vi "Module ID.vi"(11 "Config Monitor Module in":refnum<class "Config Monitor Module.lvclass">) -> (2 "Module ID":string)   [LabVIEW 2020, in "Volatus.lvlib" / "Config Monitor Module.lvclass"]
uses:
  Config Monitor Module.lvclass
  Config Monitor Module.lvclass/Config Monitor Module.ctl
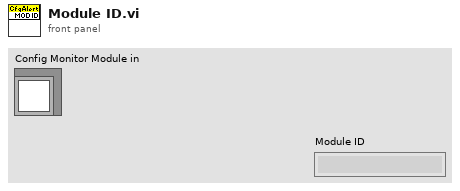
[diagram p1: front panel]
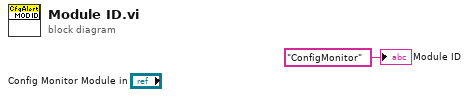
[diagram p0: block diagram]
diagram:
  "Module ID" <- "ConfigMonitor" ("Module ID")
